vi "Mail-check-login.vi"(10 "MAIL:":string, 11 "Boolean":bool) -> (3 "OK":bool)   [LabVIEW 2016]
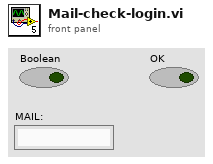
[diagram p1: front panel]
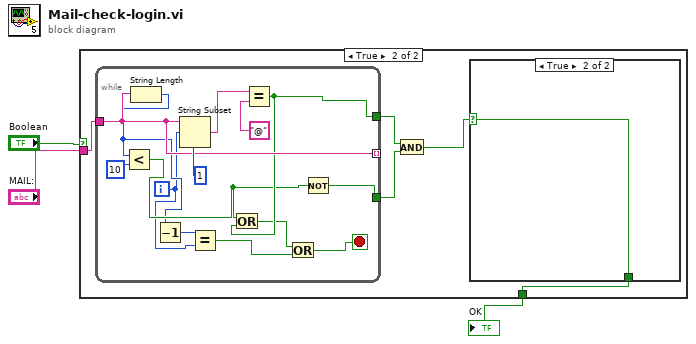
[diagram p0: block diagram]
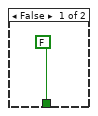
[diagram p2: hidden frame]
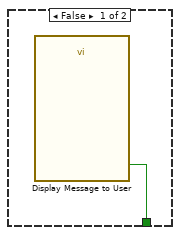
[diagram p3: hidden frame]
diagram:
  n1 = case shown="True" "Boolean" {
    tunnel: "MAIL:" -> [_ w9]
    tunnel: [FALSE ("OK") w8] -> w2
    frame False {
    }
    frame True {
      n2 = while {
        tunnel: [w18] -> w7
        tunnel: w9 -> [w20]
        tunnel: [w20] -> _ mode=indexing
        tunnel: [w16] -> w6
        i -> [w13]
        stop <- w10 stop-if-true
        n3 = String Length(string=w20) -> (length=w14:i32)
        n4 = Less?(x=w14, y=10) -> (x < y?=w17:bool)
        n5 = Decrement(x=w14) -> (x-1=w15:i32)
        n6 = String Subset(string=w20, offset (0)=w13, length (rest)=1 ("length (rest)")) -> (substring=w21:string)
        n7 = Equal?(x=w15, y=w13) -> (x = y?=w11:bool)
        n8 = Equal?(x=w21, y="@") -> (x = y?=w18:bool)
        n9 = Or(x=w17, y=w18) -> (x .or. y?=w12:bool)
        n10 = Or(x=w12, y=w11) -> (x .or. y?=w10:bool)
        n11 = Not(x=w17) -> (.not. x?=w16:bool)
      }
      n12 = And(x=w7, y=w6) -> (x .and. y?=w5:bool)
      n13 = case shown="True" w5 {
        selector: w5 -> [_ w25]
        tunnel: [w24 w25] -> w8
        frame False {
          n14 = call "Display Message to User"() -> ("OK"=w24:bool)  [unwired: 10 in, 1 out]
        }
        frame True {
        }
      }
    }
  }
  "OK" <- w2
